vi "SRV_Init_TCP Comm Loop.vi"(8 "error in (no error)":errorcluster, 11 "System Config File Path in":path) -> (0 "error out":errorcluster, 1 "Cancelled?":bool, 2 "SRV IP Address out":string, 3 "connection ID":refnum<k5>)   [LabVIEW 2014]
uses:
  Support/SRV_Command-Data Queue Data Type.ctl
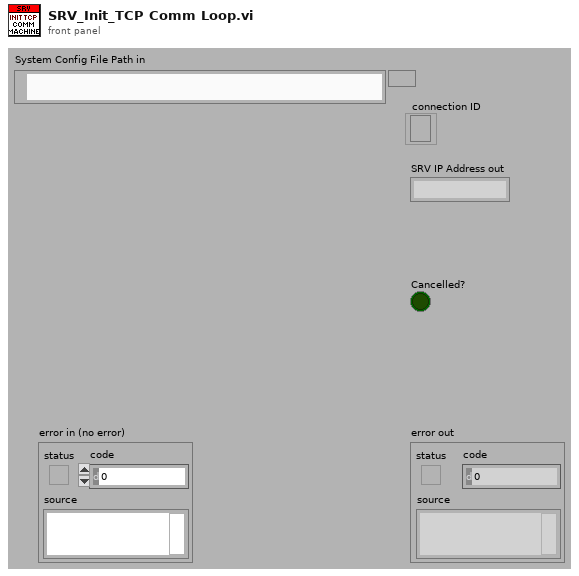
[diagram p1: front panel]
types:
  T1 = cluster{"SRV IP Address":string, "connection ID":refnum<k5>, "Cancelled?":bool, "System Config File Path":path}
  T2 = typedef "SRV_Command-Data Queue Data Type.ctl" = cluster{"Command":string, "Data":variant}
  T3 = typedef "SRV_System Config.ctl" = cluster{"SRV IP Address":string, "Video Stream Rate Period (ms)":u32, "Enable Diagnostic Log":bool, "Watchdog 1 Config":T4, "Watchdog 2 Config":T4, "Sensor Window Filepath":path}
  T4 = typedef "SRV_Watchdog Config Cluster.ctl" = cluster{"Watchdog Name":string, "Watchdog Period (s)":dbl, "Watchdog Command":T5}
  T5 = typedef "SRV_Motor Control Command Config.ctl" = cluster{"I2C Address":u8, "Register":u8, "Value":u8, "Active":bool}
  T6 = enum16{"Left Button", "Center Button", "Right Button", "Window Close"}
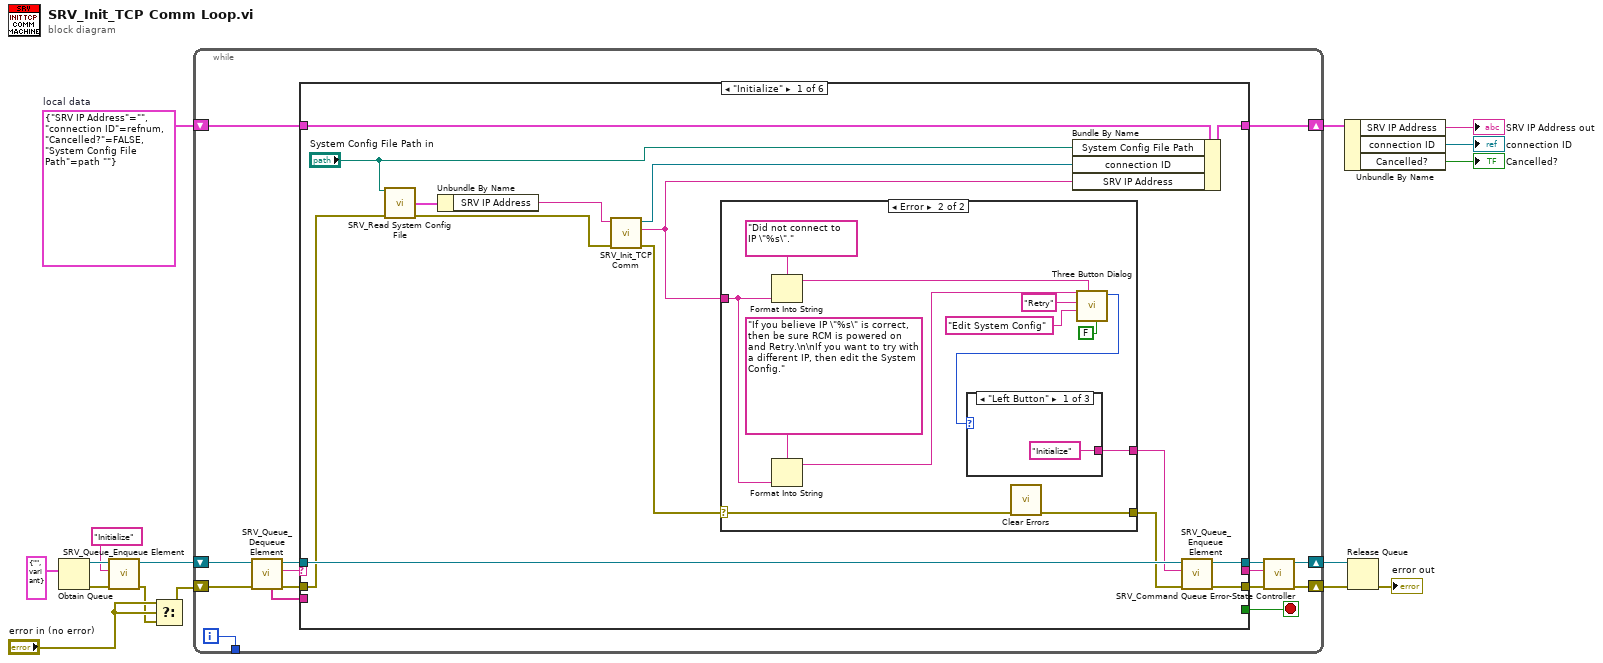
[diagram p0: block diagram]
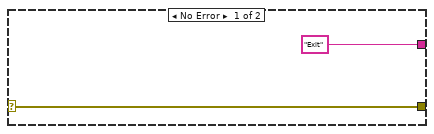
[diagram p2: hidden frame]
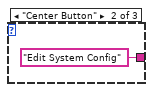
[diagram p3: hidden frame]
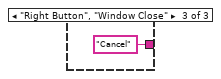
[diagram p4: hidden frame]
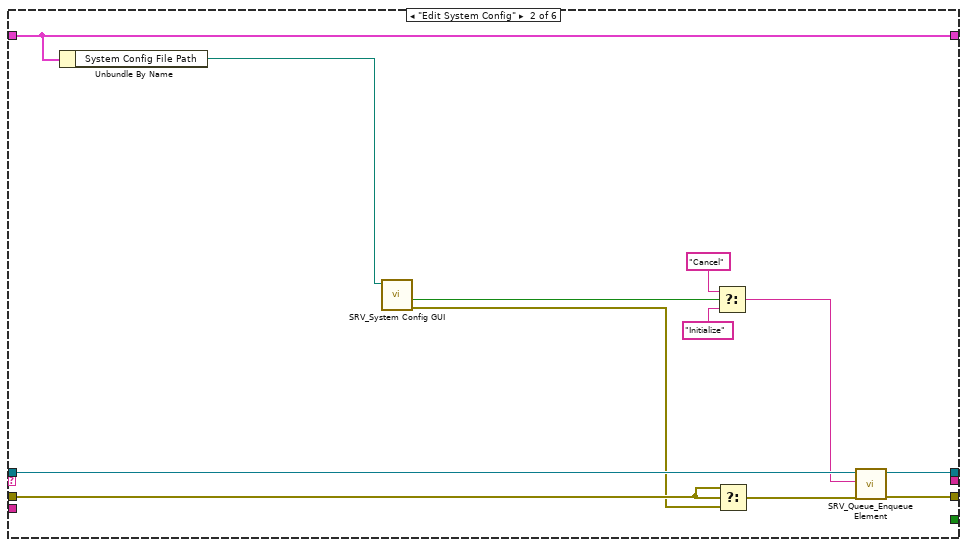
[diagram p5: hidden frame]
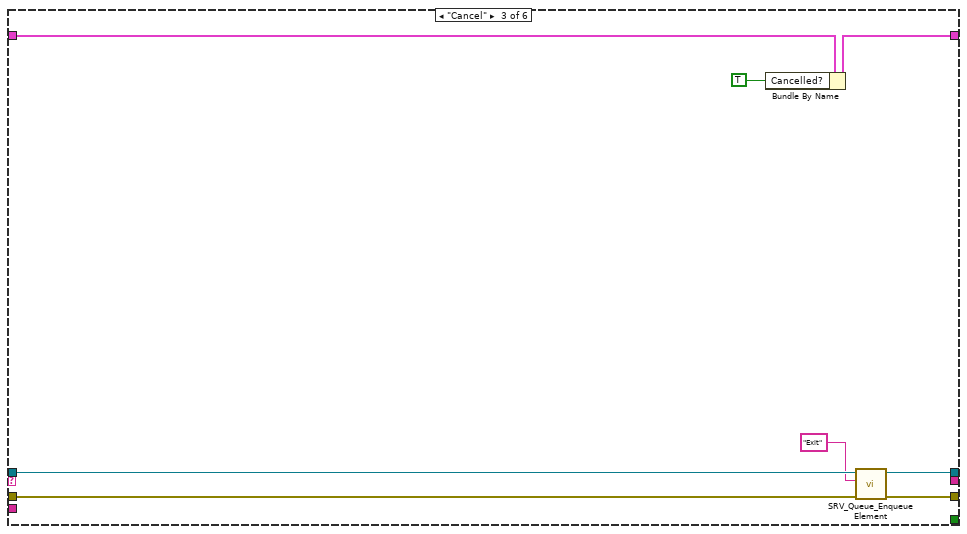
[diagram p6: hidden frame]
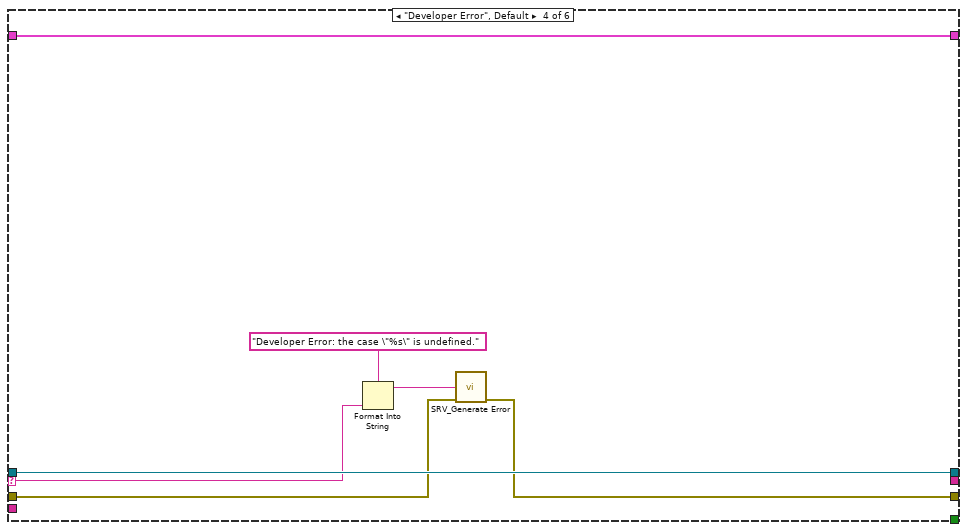
[diagram p7: hidden frame]
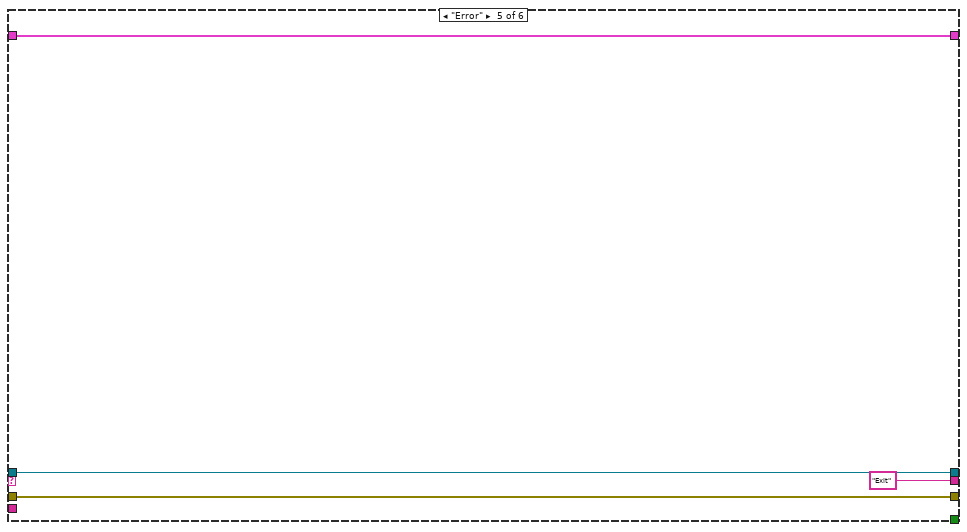
[diagram p8: hidden frame]
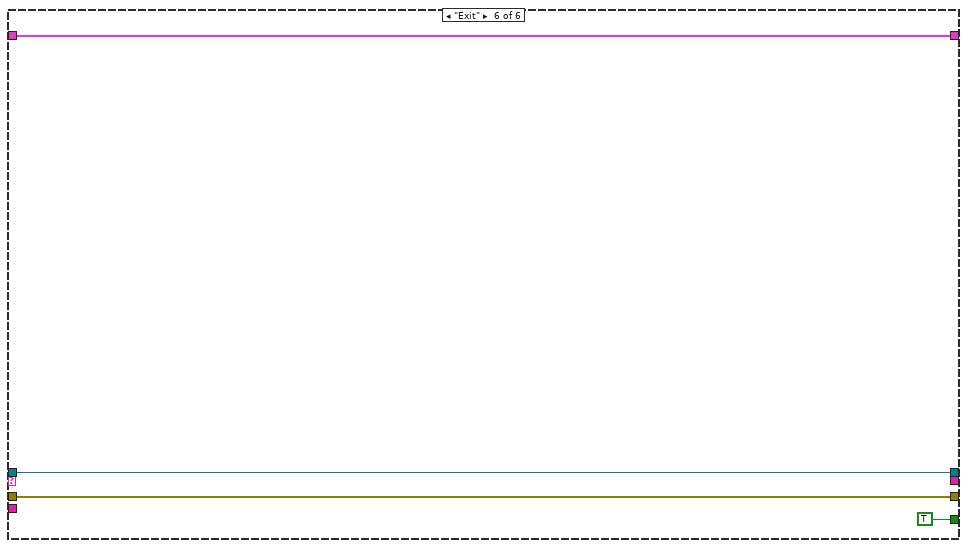
[diagram p9: hidden frame]
diagram:
  w8 = T1 {"SRV IP Address"="", "connection ID"=refnum, "Cancelled?"=FALSE, "System Config File Path"=path ""}  # local data
  n1 = Obtain Queue(element data type=T2 {"Command"="", "Data"=variant} ("Queue Data Type")) -> (queue out=w15:refnum<queue>, error out=w13:errorcluster)  [unwired: 4 in, 1 out]
  n2 = call "SRV_Queue_Enqueue Element.vi"("error in (no error)"=w13, "Command"="Initialize", "Command-Data Queue"=w15) -> ("error out"=w2:errorcluster, "Command-Data Queue out"=w14:refnum<queue>)  [unwired: 6 in, 1 out]
  n3 = Select(t="error in (no error)", s="error in (no error)", f=w2) -> (s? t:f=w1:errorcluster)
  n4 = while {
    shift-right: [w22] -> w10
    shift-left: w1 -> [w29]
    shift-right: [w24] -> w11
    shift-left: w14 -> [w28]
    shift-right: [w19] -> w7
    shift-left: w8 -> [w20]
    tunnel: [w17] -> _
    i -> [w17]
    stop <- w26 stop-if-true
    n5 = call "SRV_Queue_Dequeue Element.vi"("error in (no error)"=w29, "Command-Data Queue"=w28) -> ("error out"=w30:errorcluster, "Command"=w31:string, "Command-Data Queue out"=w27:refnum<queue>, "Command History"=w18:string[])  [unwired: 4 in, 2 out]
    n6 = case shown="\"Initialize\"" w31 {
      selector: w31 -> [_ _ _ w86 _ _]
      tunnel: w30 -> [w35 w72 w80 w88 w93 w97]
      tunnel: [w46 w74 w82 w89 w93 w97] -> w23
      tunnel: [w45 w75 w83 w90 w94 w98] -> w25
      tunnel: w27 -> [w44 w73 w81 w90 w94 w98]
      tunnel: [_ _ _ _ _ TRUE] -> w26
      tunnel: [_ _ _ _ "Exit" ("Error Command") _] -> w21
      tunnel: w20 -> [w43 w65 w78 w84 w91 w95]
      tunnel: [w42 w65 w77 w84 w91 w95] -> w19
      tunnel: w18 -> [_ _ _ _ _ _]
      frame "Initialize" {
        n7 = call "SRV_Read System Config File.vi"("System Config File Path"="System Config File Path in", "error in (no error)"=w35) -> ("System Config"=w32:T3, "error out"=w34:errorcluster)  [unwired: 10 in, 2 out]
        n8 = Unbundle By Name(w32) -> ("SRV IP Address"=w36:string)
        n9 = call "SRV_Init_TCP Comm.vi"("error in (no error)"=w34, "SRV IP Address"=w36) -> ("error out"=w38:errorcluster, "SRV IP Address dup"=w40:string, "connection ID"=w41:refnum<k5>)  [unwired: 7 in]
        n10 = case shown="Error" w38 {
          selector: w38 -> [w47 w51]
          tunnel: w40 -> [_ w52]
          tunnel: ["Exit" ("Command") w53] -> w39
          tunnel: [w47 w50] -> w37
          frame No Error {
          }
          frame Error {
            n11 = Format Into String(format string="Did not connect to IP \"%s\".", w52) -> (resulting string=w56:string)  [unwired: 2 in, 1 out]
            n12 = Format Into String(format string="If you believe IP \"%s\" is correct, then be sure RCM is powered on and Retry.\n\nIf you want to try with a different IP, then edit the System Config.", w52) -> (resulting string=w54:string)  [unwired: 2 in, 1 out]
            n13 = call <vilib>:"Clear Errors.vi"("error in (no error)"=w51) -> ("error out"=w50:errorcluster)  [unwired: 5 in, 1 out]
            n14 = call <vilib>:"Three Button Dialog.vi"("Allow user to close window? (TRUE)"=FALSE, "Window Title (\"\")"=w56, "Center Button Text (\"No\")"="Edit System Config" ("Center Button Text (\"No\")"), "Left Button Text (\"Yes\")"="Retry" ("Left Button Text (\"Yes\")"), "message"=w54) -> ("Which Button?"=w49:T6)  [unwired: 6 in]
            n15 = case shown="\"Left Button\"" w49 {
              tunnel: ["Initialize" ("Command") "Edit System Config" ("Command") "Cancel" ("Command")] -> w53
              frame "Left Button" {
              }
              frame "Center Button" {
              }
              frame "Right Button", "Window Close" {
              }
            }
          }
        }
        n16 = Bundle By Name(cluster=w43, "System Config File Path"="System Config File Path in", "connection ID"=w41, "SRV IP Address"=w40) -> (w42:T1)
        n17 = call "SRV_Queue_Enqueue Element.vi"("error in (no error)"=w37, "Command"=w39, "Command-Data Queue"=w44) -> ("error out"=w46:errorcluster, "Command-Data Queue out"=w45:refnum<queue>)  [unwired: 6 in, 1 out]
      }
      frame "Edit System Config" {
        n18 = Unbundle By Name(w65) -> ("System Config File Path"=w64:path)
        n19 = call "SRV_System Config GUI.vi"("System Config File Path in"=w64) -> ("error out"=w70:errorcluster, "Cancelled?"=w69:bool)  [unwired: 8 in, 1 out]
        n20 = Select(t="Cancel" ("Command"), s=w69, f="Initialize" ("Command")) -> (s? t:f=w67:string)
        n21 = Select(t=w72, s=w72, f=w70) -> (s? t:f=w71:errorcluster)
        n22 = call "SRV_Queue_Enqueue Element.vi"("error in (no error)"=w71, "Command"=w67, "Command-Data Queue"=w73) -> ("error out"=w74:errorcluster, "Command-Data Queue out"=w75:refnum<queue>)  [unwired: 6 in, 1 out]
      }
      frame "Cancel" {
        n23 = Bundle By Name(cluster=w78, "Cancelled?"=TRUE) -> (w77:T1)
        n24 = call "SRV_Queue_Enqueue Element.vi"("error in (no error)"=w80, "Command"="Exit", "Command-Data Queue"=w81) -> ("error out"=w82:errorcluster, "Command-Data Queue out"=w83:refnum<queue>)  [unwired: 6 in, 1 out]
      }
      frame "Developer Error", Default {
        n25 = Format Into String(format string="Developer Error: the case \"%s\" is undefined.", w86) -> (resulting string=w87:string)  [unwired: 2 in, 1 out]
        n26 = call "SRV_Generate Error.vi"("Message"=w87, "error in (no error)"=w88) -> ("error out"=w89:errorcluster)  [unwired: 13 in]
      }
      frame "Error" {
      }
      frame "Exit" {
      }
    }
    n27 = call "SRV_Command Queue Error-State Controller.vi"("error in (no error)"=w23, "Error Command"=w21, "Command-Data Queue"=w25) -> ("error out"=w22:errorcluster, "Command-Data Queue out"=w24:refnum<queue>)  [unwired: 7 in]
  }
  n28 = Unbundle By Name(w7) -> ("SRV IP Address"=→"SRV IP Address out":string, "connection ID"=→"connection ID":refnum<k5>, "Cancelled?"=→"Cancelled?":bool)
  n29 = Release Queue(queue=w11, error in (no error)=w10) -> (error out=→"error out":errorcluster)  [unwired: 1 in, 2 out]
